vi "BAE2.vi"() -> ()   [LabVIEW 2014]
doc: "3D Sensor \n\nProduces a unit vector and angle in polar coordinates of a source afer the calculating its positions [km] in a three dimensional plane and the time interval [nsec] with respect to the origin.\n\nIt also tests the validity of the source through checksum[bool].\n\nSubVi's used: calc unit vector comp start BAE2 and calc polar angles for unit vector BAE2\n\nBeverly Abadines\nPhy 350: E2"
uses:
  E2B sol/typedefs/event cluster typedef.ctl
  E2B sol/typedefs/unit vector typedef.ctl
  E2B sol/typedefs/polar angle typedef.ctl
panel:
  out "polar angles to source":T1={"theta [degrees]"=115.52371, "phi [degrees]"=-131.28725}
  out "unit vector to source":T2={"nx"=-0.59538233, "ny"=-0.6780138, "nz"=-0.43084344}
  in  "origin signal data":T3={"position [km]"=0.0, "time [nsec]"=34077005}
  in  "z signal data":T3={"position [km]"=1077.0, "time [nsec]"=35623733}
  in  "y signal data":T3={"position [km]"=1221.0, "time [nsec]"=36836521}
  in  "x signal data":T3={"position [km]"=1535.0, "time [nsec]"=37123378}
  out "checksum":sgl=0.99990445
  out "signal valid":bool=TRUE
  in  "speed of light [m/s]":sgl=300000000.0
  # "Source Direction Calculation from Timing Data"
  # "Event Data"
  # "Source Direction"
  # "Signal Validity Check"
  # "System Parameters"
  # "Beverly Abadines\nCSUSB\nPHY 350: E2"
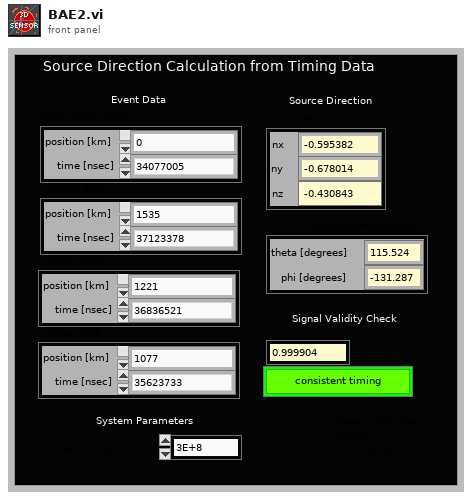
[diagram p1: front panel]
types:
  T1 = typedef "polar angle typedef.ctl" = cluster{"theta [degrees]":sgl, "phi [degrees]":sgl}
  T2 = typedef "unit vector typedef.ctl" = cluster{"nx":sgl, "ny":sgl, "nz":sgl}
  T3 = typedef "event cluster typedef.ctl" = cluster{"position [km]":sgl, "time [nsec]":i64}
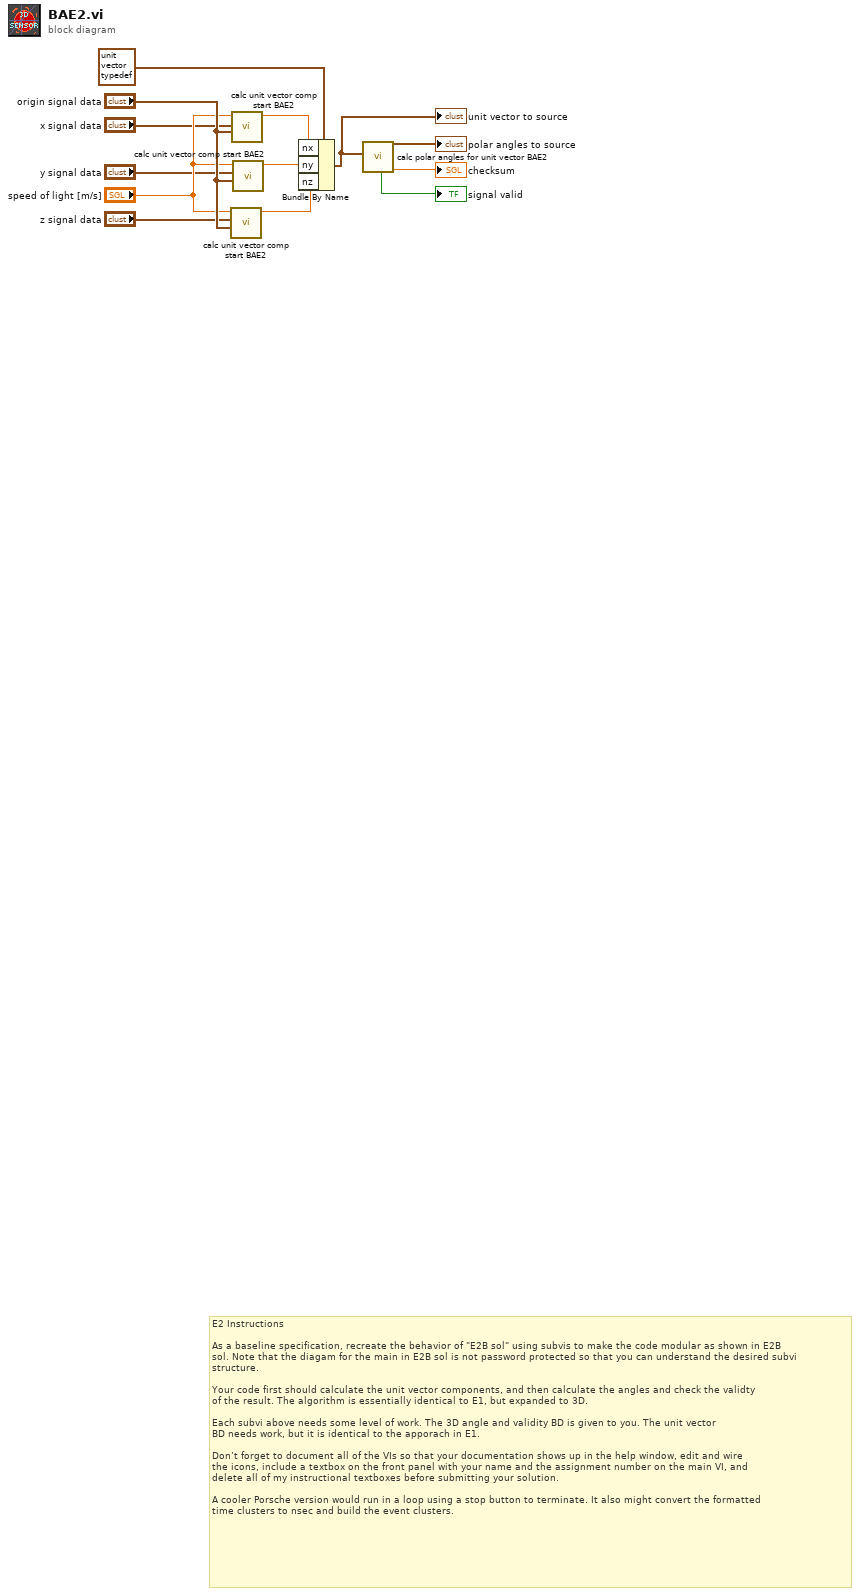
[diagram p0: block diagram]
diagram:
  # "E2 Instructions\n\nAs a baseline specification, recreate the behavior of \"E2B sol\" using subvis to make the code modular as shown in E2B \nsol. Note that the diagam for the main in E2B sol is not password protected so that you can understand the desired subvi \nstructure.\n\nYour code first should calculate the unit vector components, and then calculate the angles and check the validty\nof the result. The algorithm is essentially identical to E1, but expanded to 3D. \n\nEach subvi above needs some level of work. The 3D angle and validity BD is given to you. The unit vector\nBD needs work, but it is identical to the apporach in E1.\n\nDon’t forget to document all of the VIs so that your documentation shows up in the help window, edit and wire \nthe icons, include a textbox on the front panel with your name and the assignment number on the main VI, and \ndelete all of my instructional textboxes before submitting your solution.\n\nA cooler Porsche version would run in a loop using a stop button to terminate. It also might convert the formatted \ntime clusters to nsec and build the event clusters."
  n1 = call "calc unit vector comp start BAE2.vi"("event data at origin in"="origin signal data", "event data along axis in"="z signal data", "speed of light [m/s]"="speed of light [m/s]") -> ("component of unit vector"=w9:sgl)  [unwired: 8 in]
  n2 = call "calc unit vector comp start BAE2.vi"("event data at origin in"="origin signal data", "event data along axis in"="x signal data", "speed of light [m/s]"="speed of light [m/s]") -> ("component of unit vector"=w11:sgl)  [unwired: 8 in]
  n3 = call "calc unit vector comp start BAE2.vi"("event data at origin in"="origin signal data", "event data along axis in"="y signal data", "speed of light [m/s]"="speed of light [m/s]") -> ("component of unit vector"=w10:sgl)  [unwired: 8 in]
  n4 = Bundle By Name(cluster=T2 {"nx"=-0.59538233, "ny"=-0.6780138, "nz"=-0.43084344} ("unit vector to constant"), "nx"=w11, "ny"=w10, "nz"=w9) -> (w4:T2)
  "unit vector to source" <- w4
  n5 = call "calc polar angles for unit vector BAE2.vi"("unit vector in"=w4) -> ("signal valid"=→"signal valid":bool, "checksum"=→"checksum":sgl, "polar angles out"=→"polar angles to source":T1)  [unwired: 8 in]
